vi "receiveProgramStats.vi"(8 "error in (no error)":errorcluster, 11 "ILC in":refnum<class "ILC.lvclass">) -> (0 "error out":errorcluster, 2 "Program Stats":string, 3 "ILC out":refnum<class "ILC.lvclass">)   [LabVIEW 2015, in "ILCCommon.lvlib" / "ILC.lvclass"]
uses:
  <userlib>/Common/ILC/ILC/ILC.lvclass
  <userlib>/Common/ILC/ILC/ILC.lvclass/ILC.ctl
  <userlib>/Common/SerialProtocols/SerialCommunicator/SerialCommunicator.lvclass
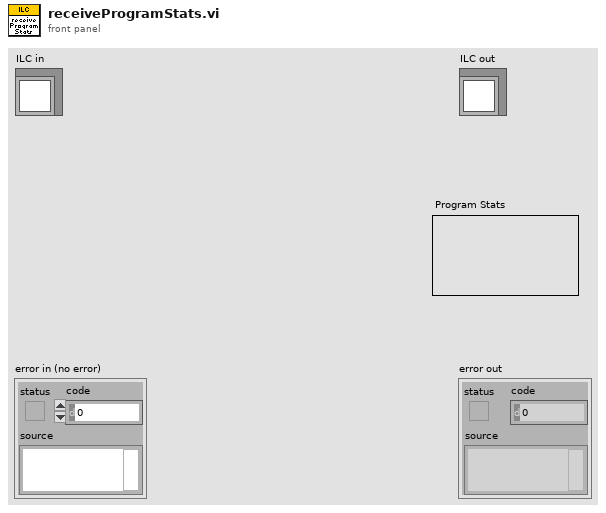
[diagram p1: front panel]
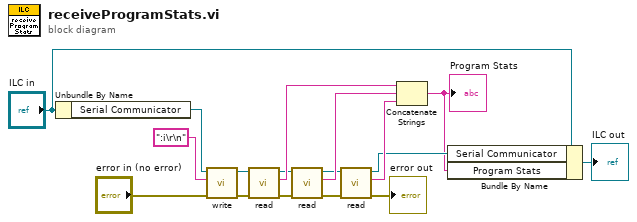
[diagram p0: block diagram]
diagram:
  n1 = Unbundle By Name("ILC in") -> ("Serial Communicator"=w11:refnum<class "SerialCommunicator.lvclass">)
  n2 = call-dynamic "write.vi"("error in (no error)"="error in (no error)", "writeString"=":i\r\n", "SerialCommunicator in"=w11) -> ("error out"=w7:errorcluster, "SerialCommunicator out"=w12:refnum<class "SerialCommunicator.lvclass">)  [unwired: 7 in]
  n3 = call-dynamic "read.vi"("error in (no error)"=w7, "SerialCommunicator in"=w12) -> ("error out"=w6:errorcluster, "stringRead"=w15:string, "SerialCommunicator out"=w13:refnum<class "SerialCommunicator.lvclass">)  [unwired: 7 in]
  n4 = call-dynamic "read.vi"("error in (no error)"=w6, "SerialCommunicator in"=w13) -> ("error out"=w5:errorcluster, "stringRead"=w16:string, "SerialCommunicator out"=w14:refnum<class "SerialCommunicator.lvclass">)  [unwired: 7 in]
  n5 = call-dynamic "read.vi"("error in (no error)"=w5, "SerialCommunicator in"=w14) -> ("error out"=→"error out":errorcluster, "stringRead"=w17:string, "SerialCommunicator out"=w4:refnum<class "SerialCommunicator.lvclass">)  [unwired: 7 in]
  n6 = Concatenate Strings(w15, w16, w17) -> (w1:string)
  "Program Stats" <- w1
  n7 = Bundle By Name(cluster="ILC in", "Serial Communicator"=w4, "Program Stats"=w1) -> (→"ILC out":refnum<class "ILC.lvclass">)
